vi "svx_SC Line Marker Position.vi"(7 "Data":T1, 11 "SC Line in":refnum<vi>) -> (1 "marker value":dbl[](array[numeric]), 2 "Marker Position":cluster{dbl, dbl}[](array[cluster]), 3 "SC Line out":refnum<vi>)   [LabVIEW 2017, in "SVX SC Line.xctl"]
uses:
  <vilib>/addons/_XControls/Shaft Centerline/SVX SC Line.xctl
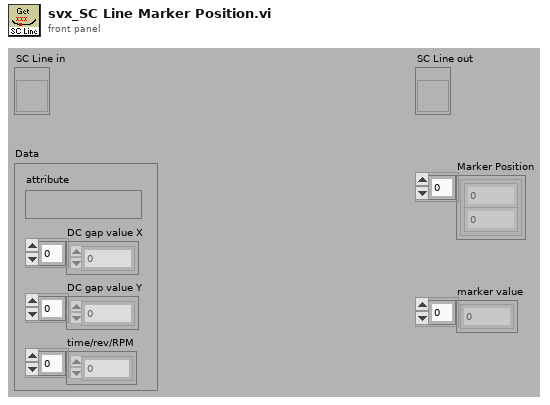
[diagram p1: front panel]
types:
  T1 = cluster{"DC gap value X":dbl[], "DC gap value Y":dbl[], "time/rev/RPM":dbl[], "attribute":variant}
  T2 = cluster{"orbit plot X":dbl[], "orbit plot Y":dbl[]}
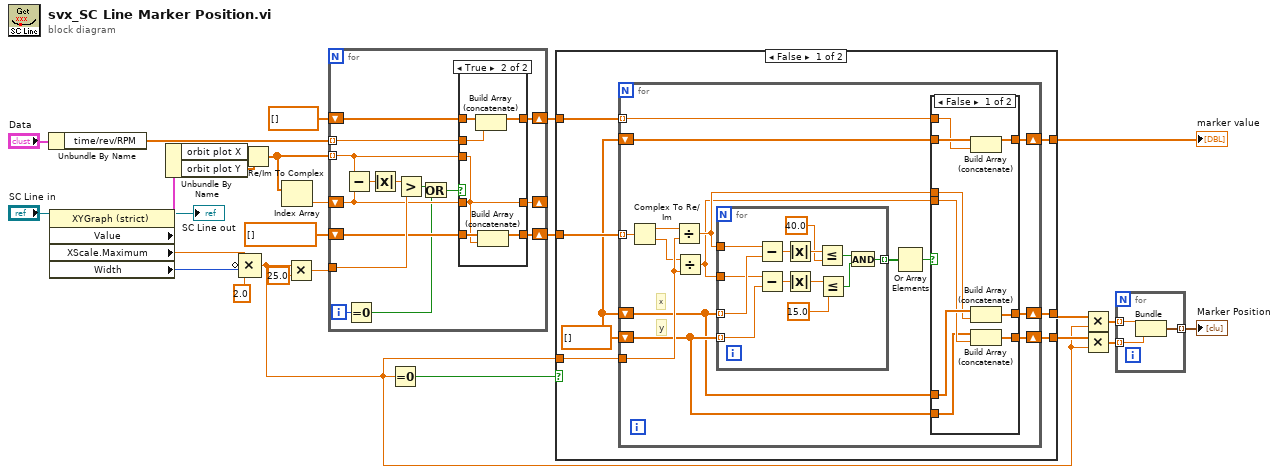
[diagram p0: block diagram]
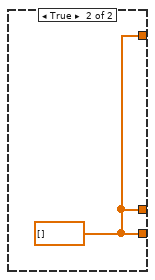
[diagram p3: hidden frame]
diagram:
  n1 = Unbundle By Name("Data") -> ("time/rev/RPM"=w15:dbl[])
  n2 = property class="XYGraph (strict)"(reference="SC Line in") -> (reference out=→"SC Line out":refnum<vi>, "Value"=w5:T2, "XScale.Maximum"=w1:dbl, "Width"=w26:u32)  [unwired: 1 in, 1 out]
  n3 = Unbundle By Name(w5) -> ("orbit plot X"=w4:dbl[], "orbit plot Y"=w3:dbl[])
  n4 = Compound Arithmetic op=MULTIPLY(w1, invert w26, 2.0 ("value")) -> (w17:dbl)
  n5 = Re/Im To Complex(1:w3, 2:w4) -> (0:w8:cdb[])
  n6 = Index Array(array=w8) -> (element=w24:cdb)  [unwired: 1 in]
  n7 = Multiply(x=w17, y=25.0) -> (x*y=w22:dbl)
  n8 = for {
    tunnel: w8 -> [w38] mode=indexing
    shift-right: [w37] -> _
    shift-left: w24 -> [w36]
    tunnel: w22 -> [w39]
    shift-right: [w34] -> w12
    shift-left: cdb[] [] ("r * e^(i*theta)") -> [w35]
    tunnel: w15 -> [w31] mode=indexing
    shift-right: [w32] -> w13
    shift-left: dbl[] [] -> [w33]
    i -> [w30]
    n9 = Subtract(x=w38, y=w36) -> (x-y=w41:cdb)
    n10 = Equal To 0?(x=w30) -> (x = 0?=w29:bool)
    n11 = Absolute Value(x=w41) -> (abs(x)=w40:dbl)
    n12 = Greater?(x=w40, y=w39) -> (0:w28:bool)
    n13 = Or(x=w28, y=w29) -> (x .or. y?=w27:bool)
    n14 = case shown="True" w27 {
      tunnel: w38 -> [_ w49]
      tunnel: [w44 w49] -> w37
      tunnel: w36 -> [w44 _]
      tunnel: w35 -> [w43 w50]
      tunnel: [w43 w48] -> w34
      tunnel: w33 -> [w42 w47]
      tunnel: [w42 w45] -> w32
      tunnel: w31 -> [_ w46]
      frame False {
      }
      frame True {
        n15 = Build Array (concatenate)(w47, w46) -> (w45:dbl[])
        n16 = Build Array (concatenate)(w50, w49) -> (w48:cdb[])
      }
    }
  }
  n17 = Equal To 0?(x=w17) -> (x = 0?=w20:bool)
  n18 = case shown="False" w20 {
    tunnel: w12 -> [w57 _]
    tunnel: w17 -> [w56 _]
    tunnel: [w55 w98] -> w19
    tunnel: [w54 w98] -> w18
    tunnel: w13 -> [w53 _]
    tunnel: [w51 w98] -> w9
    frame False {
      w52 = dbl[] []
      n19 = for {
        tunnel: w57 -> [w61] mode=indexing
        tunnel: w56 -> [w72]
        shift-right: [w67] -> w55
        shift-left: w52 -> [w68]
        shift-right: [w66] -> w54
        shift-left: w52 -> [w69]
        tunnel: w53 -> [w58] mode=indexing
        shift-right: [w60] -> w51
        shift-left: w52 -> [w59]
        # "y"
        # "x"
        n20 = Complex To Re/Im(x + iy=w61) -> (x=w65:dbl, y=w63:dbl)
        n21 = Divide(x=w65, y=w72) -> (x/y=w64:dbl)
        n22 = Divide(x=w63, y=w72) -> (x/y=w62:dbl)
        n23 = for {
          tunnel: w64 -> [w97]
          tunnel: w62 -> [w95]
          tunnel: w68 -> [w96] mode=indexing
          tunnel: w69 -> [w94] mode=indexing
          tunnel: [w85] -> w71 mode=indexing
          n24 = Subtract(x=w97, y=w96) -> (x-y=w93:dbl)
          n25 = Subtract(x=w95, y=w94) -> (x-y=w92:dbl)
          n26 = Absolute Value(x=w93) -> (abs(x)=w91:dbl)
          n27 = Absolute Value(x=w92) -> (abs(x)=w90:dbl)
          n28 = Less Or Equal?(x=w91, y=40.0) -> (x <= y?=w87:bool)
          n29 = Less Or Equal?(x=w90, y=15.0) -> (x <= y?=w86:bool)
          n30 = And(x=w87, y=w86) -> (x .and. y?=w85:bool)
        }
        n31 = Or Array Elements(Boolean array=w71) -> (logical OR=w70:bool)
        n32 = case shown="False" w70 {
          tunnel: w64 -> [w79 _]
          tunnel: w62 -> [w77 _]
          tunnel: w69 -> [w76 w83]
          tunnel: w68 -> [w81 w84]
          tunnel: [w80 w84] -> w67
          tunnel: [w78 w83] -> w66
          tunnel: [w75 w82] -> w60
          tunnel: w59 -> [w74 w82]
          tunnel: w58 -> [w73 _]
          frame False {
            n33 = Build Array (concatenate)(w74, w73) -> (w75:dbl[])
            n34 = Build Array (concatenate)(w81, w79) -> (w80:dbl[])
            n35 = Build Array (concatenate)(w76, w77) -> (w78:dbl[])
          }
          frame True {
            # "overlap"
          }
        }
      }
    }
    frame True {
      w98 = dbl[] []
    }
  }
  "marker value" <- w9
  n36 = Multiply(x=w19, y=w17) -> (x*y=w10:dbl[])
  n37 = Multiply(x=w18, y=w17) -> (x*y=w11:dbl[])
  n38 = for {
    tunnel: w10 -> [w101] mode=indexing
    tunnel: w11 -> [w100] mode=indexing
    tunnel: [w99] -> w16 mode=indexing
    n39 = Bundle(w101, w100) -> (w99:cluster{dbl, dbl})  [unwired: 1 in]
  }
  "Marker Position" <- w16
